vi "ReadExcelWIP.vi"(6 "Element":string) -> (0 "error out":errorcluster, 3 "element":string)   [LabVIEW 2012]
doc: "Before runnig this vi you need to select the sheet and the cell you want to retrieve in LabVIEW. When you start this vi, LabVIEW will ask you the name of the Excel file. This vi was written with Excel from MS Office 97. If you edit this VI and do not have this exact version of Excel registered correctly you will get a broken arrow due to the difference in ActiveX method among Excel version. Make sure you make a copy of this vi before editing it."
uses:
  C:/Users/yy/Downloads/Search 2D Array 2009/Search 2D Array 2009/Search 2D Array (String).vi
panel:
  out "Locations":i32[][](array[numeric])
  out "transposed array":string[][](array[string])
  out "data":string[][](array[string])
  in  "end cell":string="h8192"
  in  "start cell":string="d5"
  in  "sheet#":i32=1
  in  "Path":path=path "E:/m100/data/wip-0929.xls"
  in  "Excel._Worksheet":refnum<k7>
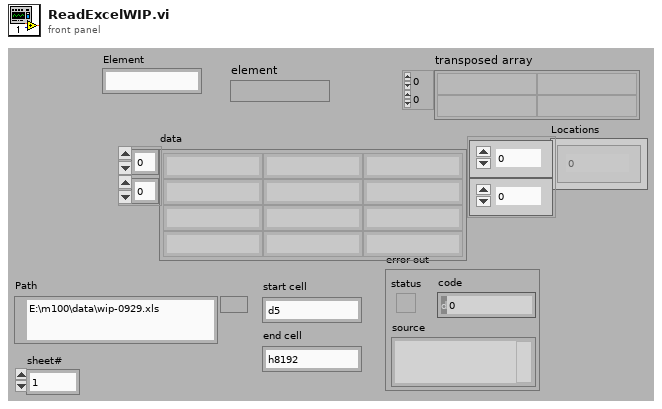
[diagram p1: front panel]
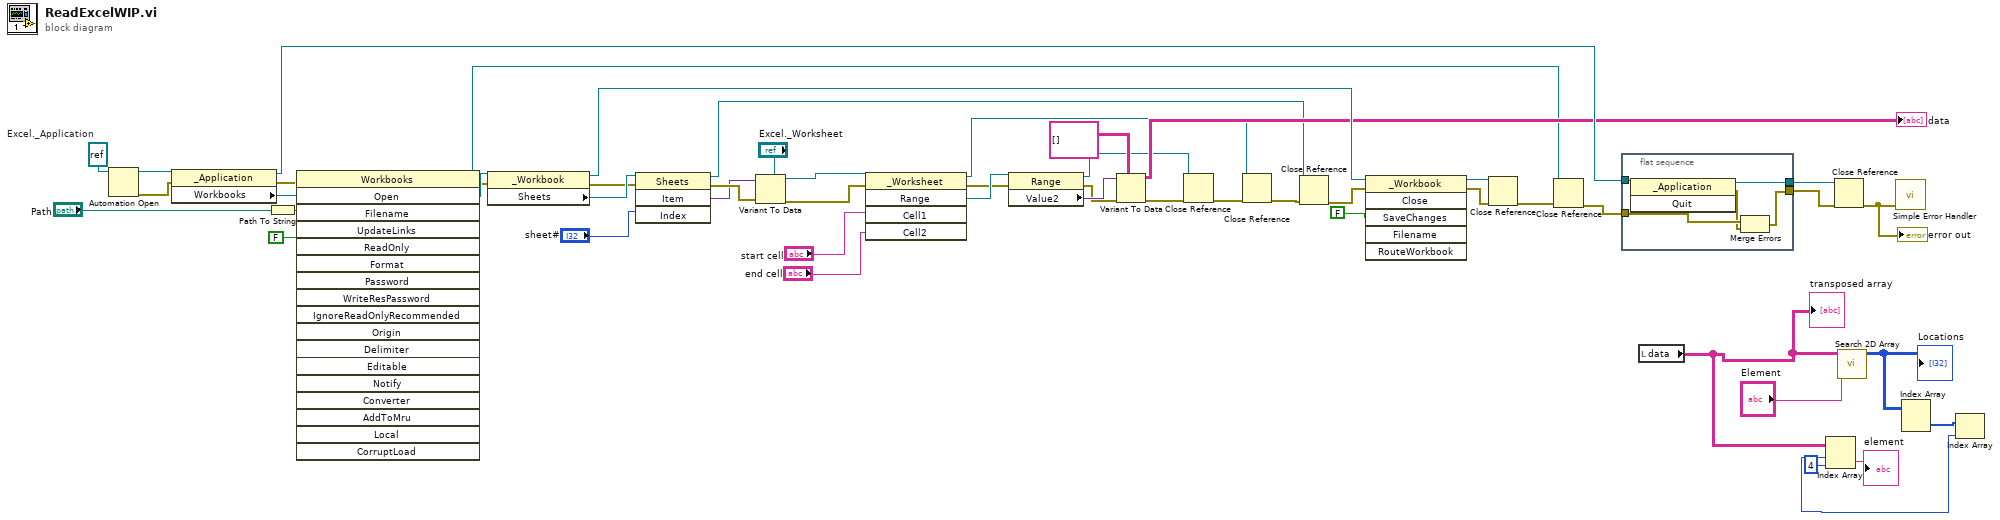
[diagram p0: block diagram]
diagram:
  w18 = refnum<k7> refnum  # Excel._Application
  n1 = Automation Open(Automation Refnum=w18) -> (Automation Refnum=w32:refnum<k7>, error out=w50:errorcluster)  [unwired: 3 in]
  n2 = property class="_Application"(reference=w32, error in=w50) -> (reference out=w22:refnum<k7>, error out=w48:errorcluster, "Workbooks"=w49:refnum<k7>)
  n3 = Path To String(path="Path") -> (string=w35:string)
  n4 = invoke class="Workbooks" method="Open"(reference=w49, error in=w48, "Filename"=w35, "ReadOnly"=FALSE) -> (reference out=w8:refnum<k7>, error out=w46:errorcluster, "Open"=w47:refnum<k7>)  [unwired: 14 in, 15 out]
  n5 = property class="_Workbook"(reference=w47, error in=w46) -> (reference out=w29:refnum<k7>, error out=w33:errorcluster, "Sheets"=w45:refnum<k7>)
  n6 = invoke class="Sheets" method="Item"(reference=w45, error in=w33, "Index"="sheet#") -> (reference out=w9:refnum<k7>, error out=w44:errorcluster, "Item"=w43:variant)  [unwired: 1 in, 1 out]
  n7 = Variant To Data(error in=w44, type="Excel._Worksheet", Variant=w43) -> (data=w42:refnum<k7>, error out=w41:errorcluster)
  n8 = invoke class="_Worksheet" method="Range"(reference=w42, error in=w41, "Cell1"="start cell", "Cell2"="end cell") -> (reference out=w11:refnum<k7>, error out=w39:errorcluster, "Range"=w40:refnum<k7>)  [unwired: 1 in, 2 out]
  n9 = property class="Range"(reference=w40, error in=w39) -> (reference out=w10:refnum<k7>, error out=w37:errorcluster, "Value2"=w38:variant)
  n10 = Variant To Data(error in=w37, type=string[][] [], Variant=w38) -> (data=→"data":string[][], error out=w36:errorcluster)
  n11 = Close Reference(reference=w10, error in (no error)=w36) -> (error out=w31:errorcluster)
  n12 = Close Reference(reference=w11, error in (no error)=w31) -> (error out=w30:errorcluster)
  n13 = Close Reference(reference=w9, error in (no error)=w30) -> (error out=w28:errorcluster)
  n14 = invoke class="_Workbook" method="Close"(reference=w29, error in=w28, "SaveChanges"=FALSE) -> (reference out=w26:refnum<k7>, error out=w27:errorcluster)  [unwired: 3 in, 4 out]
  n15 = Close Reference(reference=w26, error in (no error)=w27) -> (error out=w25:errorcluster)
  n16 = Close Reference(reference=w8, error in (no error)=w25) -> (error out=w24:errorcluster)
  n17 = flat-sequence {
    tunnel: w24 -> [w54]
    tunnel: [w52] -> w23
    tunnel: w22 -> [w56]
    tunnel: [w55] -> w21
    frame #0 {
      n18 = invoke class="_Application" method="Quit"(reference=w56) -> (reference out=w55:refnum<k7>, error out=w53:errorcluster)  [unwired: 2 in, 1 out]
      n19 = Merge Errors(w54, w53) -> (w52:errorcluster)
    }
  }
  n20 = local read "data"() -> (w7:string[][])
  "transposed array" <- w7
  n21 = Close Reference(reference=w21, error in (no error)=w23) -> (error out=w20:errorcluster)
  "error out" <- w20
  n22 = call-poly "Search 2D Array.vi"("Element"="Element", "Array"=w7) -> ("Locations"=w6:i32[][])  [unwired: 9 in]
  "Locations" <- w6
  n23 = call <vilib>:"Simple Error Handler.vi"("error in (no error)"=w20) -> ()  [unwired: 4 in, 5 out]
  n24 = Index Array(array=w6) -> (element=w5:i32[])  [unwired: 2 in]
  n25 = Index Array(array=w5) -> (element=w3:i32)  [unwired: 1 in]
  n26 = Index Array(array=w7, index (row)=w3, index (col)=4 ("disabled index (col)")) -> (element=→"element":string)
